vi "Data_Cluster_To_Mixed_signals.vi"(8 "error in (no error)":errorcluster, 11 "Data in":T2) -> (0 "error out":errorcluster, 3 "Data out":T1)   [LabVIEW 2013]
uses:
  Kontrolki/Przetwarzanie/Kanaly.ctl
  <vilib>/Waveform/DWDTOps.llb/DWDT Boolean Array to Digital.vi
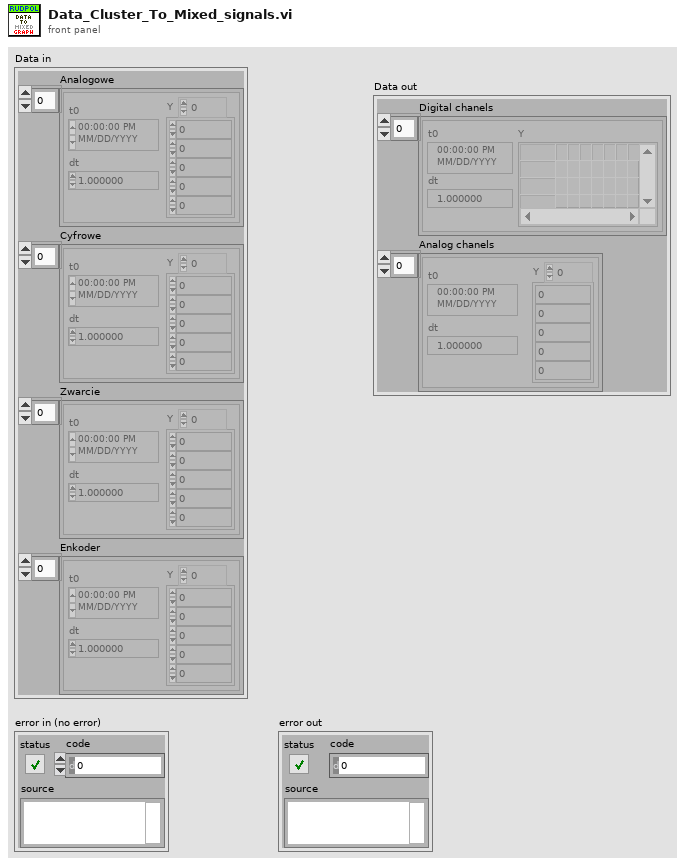
[diagram p1: front panel]
types:
  T1 = cluster{"Digital chanels":digitalwaveform[], "Analog chanels":waveform(dbl)[]}
  T2 = typedef "Kanaly.ctl" = cluster{"Analogowe":waveform(dbl)[], "Cyfrowe":waveform(dbl)[], "Zwarcie":waveform(dbl)[], "Enkoder":waveform(dbl)[]}
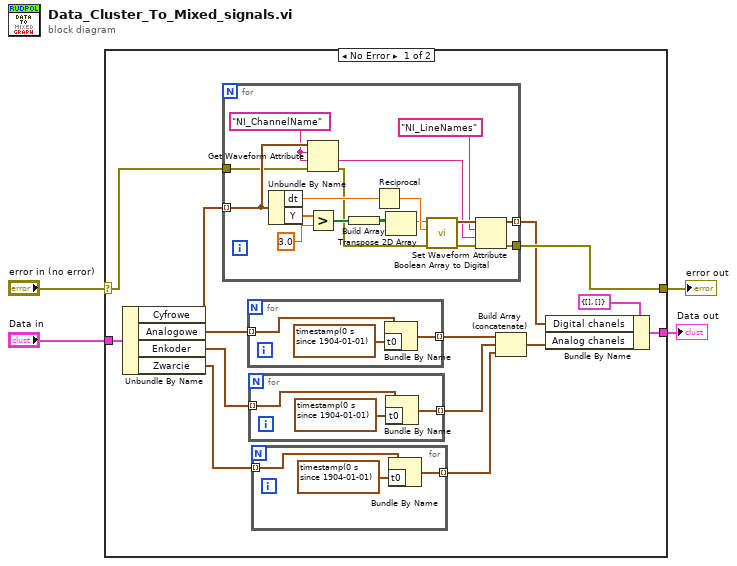
[diagram p0: block diagram]
diagram:
  n1 = case shown="No Error" "error in (no error)" {
    selector: "error in (no error)" -> [w6 w45]
    tunnel: "Data in" -> [w18 _]
    tunnel: [w7 _] -> w1
    tunnel: [w13 w45] -> w4
    frame No Error {
      n2 = Unbundle By Name(w18) -> ("Cyfrowe"=w17:waveform(dbl)[], "Analogowe"=w16:waveform(dbl)[], "Enkoder"=w15:waveform(dbl)[], "Zwarcie"=w14:waveform(dbl)[])
      n3 = for {
        tunnel: w17 -> [w43] mode=indexing
        tunnel: [w31] -> w9 mode=indexing
        tunnel: [w30] -> w13
        tunnel: w6 -> [w28]
        w42 = "NI_ChannelName" ("name")
        n4 = Unbundle By Name(w43) -> ("dt"=w34:dbl, "Y"=w44:dbl[])
        n5 = Get Waveform Attribute(4:w28, 5:w42, 6:w42, 7:w43) -> (0:w29:errorcluster, 1:w32:string)  [unwired: 2 out]
        n6 = Greater?(x=w44, y=3.0) -> (0:w36:bool[])
        n7 = Build Array(w36) -> (w37:bool[][])
        n8 = Reciprocal(x=w34) -> (1/x=w41:dbl)
        n9 = Transpose 2D Array(2D array=w37) -> (transposed array=w38:bool[][])
        n10 = call-poly <vilib>:"Boolean Array to Digital.vi"("error in (no error)"=w29, "sample rate"=w41, "boolean array"=w38) -> ("error out"=w39:errorcluster, "digital waveform"=w40:digitalwaveform)  [unwired: 7 in]
        n11 = Set Waveform Attribute(4:w39, 5:w32, 6:"NI_LineNames" ("name"), 7:w40) -> (0:w30:errorcluster, 3:w31:digitalwaveform)  [unwired: 1 out]
      }
      n12 = for {
        tunnel: w16 -> [w27] mode=indexing
        tunnel: [w25] -> w12 mode=indexing
        n13 = Bundle By Name(cluster=w27, "t0"=timestamp(0 s since 1904-01-01)) -> (w25:waveform(dbl))
      }
      n14 = for {
        tunnel: w15 -> [w24] mode=indexing
        tunnel: [w22] -> w11 mode=indexing
        n15 = Bundle By Name(cluster=w24, "t0"=timestamp(0 s since 1904-01-01)) -> (w22:waveform(dbl))
      }
      n16 = for {
        tunnel: w14 -> [w21] mode=indexing
        tunnel: [w19] -> w5 mode=indexing
        n17 = Bundle By Name(cluster=w21, "t0"=timestamp(0 s since 1904-01-01)) -> (w19:waveform(dbl))
      }
      n18 = Build Array (concatenate)(w12, w11, w5) -> (w8:waveform(dbl)[])
      n19 = Bundle By Name(cluster=T1 {"Digital chanels"=[], "Analog chanels"=[]}, "Digital chanels"=w9, "Analog chanels"=w8) -> (w7:T1)
    }
    frame Error {
      # "#todo zlikwidowaæ wartoœæ domyœln¹"
    }
  }
  "error out" <- w4
  "Data out" <- w1
